vi "_Update Parameter List.vi"(6 "Data":dbl, 7 "Channel ID":string="203", 8 "error in (no error)":errorcluster, 10 "Experiment Node":refnum<k20>, 11 "DOM Document":refnum<k20>) -> (0 "error out":errorcluster, 2 "Experiment Node out":refnum<k20>, 3 "DOM Document out":refnum<k20>)   [LabVIEW 2012]
uses:
  <vilib>/xml/Close Reference(Node).vi
  <vilib>/xml/NI_XML.lvlib
  <resource>/objmgr/DOMUserDefRef.rc
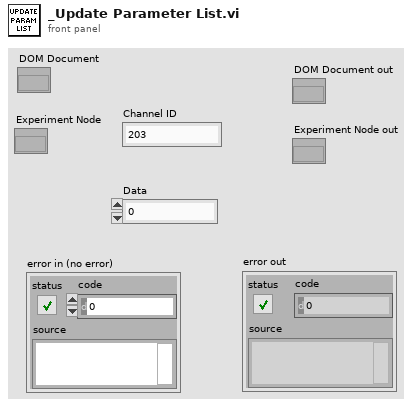
[diagram p1: front panel]
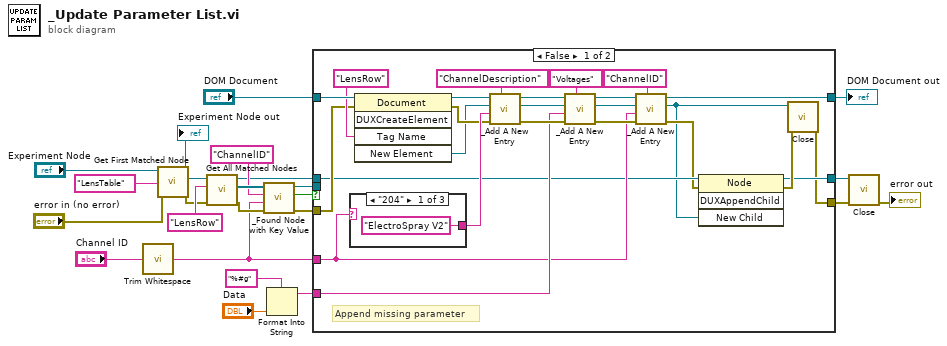
[diagram p0: block diagram]
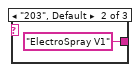
[diagram p2: hidden frame]
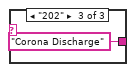
[diagram p3: hidden frame]
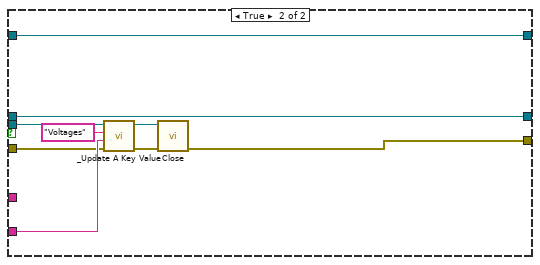
[diagram p4: hidden frame]
diagram:
  n1 = call <vilib>:"Trim Whitespace.vi"("string"="Channel ID") -> ("trimmed string"=w3:string)  [unwired: 1 in]
  n2 = call <vilib>:"Get First Matched Node.vi"("error in (no error)"="error in (no error)", "XPath expression"="LensTable", "node in"="Experiment Node") -> ("error out"=w19:errorcluster, "node result"=w20:refnum<k20>, "node out"=→"Experiment Node out":refnum<k20>)  [unwired: 6 in]
  n3 = call <vilib>:"Get All Matched Nodes.vi"("error in (no error)"=w19, "XPath expression"="LensRow", "node in"=w20) -> ("error out"=w15:errorcluster, "node result array"=w17:refnum<k20>[], "node out"=w4:refnum<k20>)  [unwired: 6 in]
  n4 = call "_Found Node with Key Value.vi"("error in (no error)"=w15, "Value"=w3, "Key"="ChannelID", "nodes"=w17) -> ("error out"=w10:errorcluster, "Found"=w13:bool, "node out"=w12:refnum<k20>)  [unwired: 1 in]
  n5 = Format Into String(format string="%#g", "Data") -> (resulting string=w11:string)  [unwired: 2 in, 1 out]
  n6 = case shown="False" w13 {
    tunnel: w12 -> [_ w61]
    tunnel: w11 -> [w34 w59]
    tunnel: w10 -> [w47 w58]
    tunnel: [w25 w55] -> w9
    tunnel: "DOM Document" -> [w49 w54]
    tunnel: w3 -> [w33 _]
    tunnel: w4 -> [w31 w53]
    tunnel: [w27 w54] -> w2
    tunnel: [w26 w53] -> w1
    frame False {
      # "Append missing parameter"
      n7 = case shown="\"204\"" w33 {
        tunnel: ["ElectroSpray V2" ("Data") "ElectroSpray V1" ("Data") "Corona Discharge" ("Data")] -> w45
        frame "204" {
        }
        frame "203", Default {
        }
        frame "202" {
        }
      }
      n8 = invoke class="Document" method="DUXCreateElement"(reference=w49, error in=w47, "Tag Name"="LensRow") -> (reference out=w36:refnum<k20>, error out=w35:errorcluster, "New Element"=w32:refnum<k20>)  [unwired: 2 in, 2 out]
      n9 = call "_Add A New Entry.vi"("Tag Name"="ChannelDescription", "error in (no error)"=w35, "Data"=w45, "Parent Node"=w32, "DOM document"=w36) -> ("error out"=w41:errorcluster, "Parent Node out"=w40:refnum<k20>, "DOM document out"=w42:refnum<k20>)  [unwired: 1 in]
      n10 = call "_Add A New Entry.vi"("Tag Name"="Voltages", "error in (no error)"=w41, "Data"=w34, "Parent Node"=w40, "DOM document"=w42) -> ("error out"=w37:errorcluster, "Parent Node out"=w38:refnum<k20>, "DOM document out"=w39:refnum<k20>)  [unwired: 1 in]
      n11 = call "_Add A New Entry.vi"("Tag Name"="ChannelID", "error in (no error)"=w37, "Data"=w33, "Parent Node"=w38, "DOM document"=w39) -> ("error out"=w30:errorcluster, "Parent Node out"=w28:refnum<k20>, "DOM document out"=w27:refnum<k20>)  [unwired: 1 in]
      n12 = invoke class="Node" method="DUXAppendChild"(reference=w31, error in=w30, "New Child"=w28) -> (reference out=w26:refnum<k20>, error out=w29:errorcluster)  [unwired: 1 in, 2 out]
      n13 = call-poly <vilib>:"Close.vi"("error in (no error)"=w29, "node"=w28) -> ("error out"=w25:errorcluster)  [unwired: 7 in]
    }
    frame True {
      n14 = call "_Update A Key Value.vi"("error in (no error)"=w58, "Value"=w59, "Key"="Voltages", "node in"=w61) -> ("error out"=w57:errorcluster, "node out"=w56:refnum<k20>)  [unwired: 2 in]
      n15 = call-poly <vilib>:"Close.vi"("error in (no error)"=w57, "node"=w56) -> ("error out"=w55:errorcluster)  [unwired: 7 out]
    }
  }
  "DOM Document out" <- w2
  n16 = call-poly <vilib>:"Close.vi"("error in (no error)"=w9, "node"=w1) -> ("error out"=→"error out":errorcluster)  [unwired: 7 out]
